vi "GetSlideScaleVisible.vi"(9 "Scale":refnum<class "Scale.lvclass">) -> (3 "Scale out":refnum<class "Scale.lvclass">, 4 "scale visible":bool)   [LabVIEW 2014, in "Raspberry Pi Compatible Compiler for LabVIEW.lvlib" / "PythonConverter_GUI.lvclass"]
uses:
  PythonConverter_GUI.lvclass
  VI Interpreter/Classes/Scale/Scale.lvclass
  VI Interpreter/Classes/Scale/Scale.lvclass/Scale.ctl
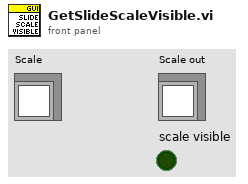
[diagram p1: front panel]
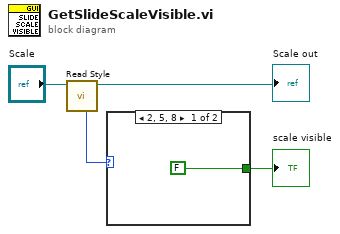
[diagram p0: block diagram]
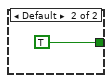
[diagram p2: hidden frame]
diagram:
  n1 = call "Read Style.vi"("Scale in"="Scale") -> ("Scale out"=→"Scale out":refnum<class "Scale.lvclass">, "Style"=w2:u8)  [unwired: 7 in]
  n2 = case shown="2, 5, 8" w2 {
    tunnel: [FALSE TRUE] -> w1
    frame 2, 5, 8 {
    }
    frame Default {
    }
  }
  "scale visible" <- w1
